vi "Obtain Request Events.vi"(8 "error in (no error)":errorcluster, 10 "Create New? (F)":bool) -> (0 "error out":errorcluster, 2 "Navigation Request Events":T1)   [LabVIEW 2022 SP3, in "Navigation.lvlib"]
doc: "This VI Obtains/Creates the Requests events that will be used for other modules to communicate with the module that owns this VI. These Requests events will be accessed only via Public API methods for this module.\n\n<b>NOTE</b>: The contents of this VI are automatically generated and modified by the <b>Tools > Delacor > DQMH</b> utilities. Consider using those utilities instead of making your own modifications to this VI.\n____\nHAMPEL SOFTWARE ENGINEERING v2.6.0 (2023-12-19 10:54)"
uses:
  Navigation.lvlib
  Request Events--cluster.ctl
  Stop Argument--cluster.ctl
  Show Panel Argument--cluster.ctl
  Hide Panel Argument--cluster.ctl
  Get Module Execution Status Argument--cluster.ctl
  Show Diagram Argument--cluster.ctl
  Prepare Argument--cluster.ctl
  Update Navigation Argument--cluster.ctl
  Sub-VIs/Ctl Target.ctl
  Configure Argument--cluster.ctl
  Select Listbox Element Argument--cluster.ctl
  Set Visibility Argument--cluster.ctl
  Sub-VIs/Visibility options--enum.ctl
  Set Disabled State Argument--cluster.ctl
panel:
  # "NOTE: The contents of this VI are automatically generated and modified by the Tools > Delacor > DQMH utilities. Consider using those utilities instead of making your own modifications to this VI."
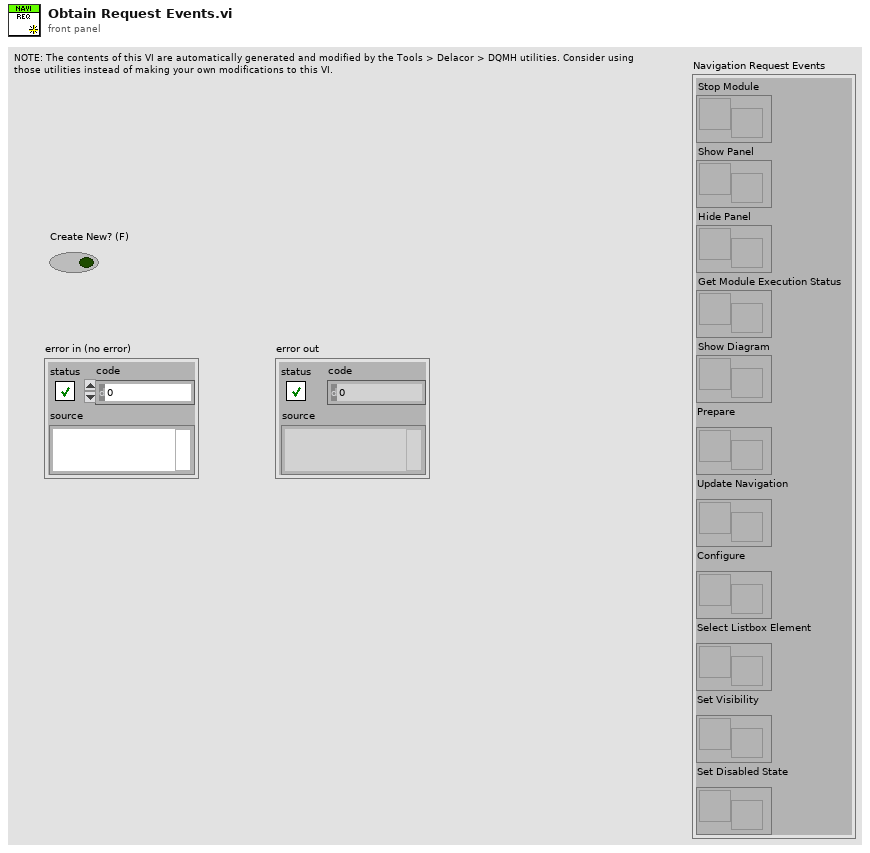
[diagram p1: front panel]
types:
  T1 = typedef "Navigation.lvlib/Request Events--cluster.ctl" = cluster{"Stop Module":refnum<user-event>, "Show Panel":refnum<user-event>, "Hide Panel":refnum<user-event>, "Get Module Execution Status":refnum<user-event>, "Show Diagram":refnum<user-event>, "Prepare":refnum<user-event>, "Update Navigation":refnum<user-event>, "Configure":refnum<user-event>, "Select Listbox Element":refnum<user-event>, "Set Visibility":refnum<user-event>, "Set Disabled State":refnum<user-event>}
  T2 = typedef "Navigation.lvlib/Set Disabled State Argument--cluster.ctl" = cluster{"Control Name":string, "Control State":enum8{"Enabled", "Disabled", "Disabled and Grayed Out"}}
  T3 = typedef "Navigation.lvlib/Set Visibility Argument--cluster.ctl" = cluster{"Control Name":string, "Visibility":T4}
  T4 = typedef "Navigation.lvlib/Visibility options--enum.ctl" = enum16{"visible", "hidden"}
  T5 = typedef "Navigation.lvlib/Select Listbox Element Argument--cluster.ctl" = cluster{"Name":string, "Index":i32}
  T6 = typedef "Navigation.lvlib/Configure Argument--cluster.ctl" = cluster{"Boolean":bool}
  T7 = typedef "Navigation.lvlib/Update Navigation Argument--cluster.ctl" = cluster{"Ctl Target":T8, "Name":string, "Data":variant}
  T8 = typedef "Navigation.lvlib/Ctl Target.ctl" = enum16{"Top Button", "Sub ListBox"}
  T9 = typedef "Navigation.lvlib/Prepare Argument--cluster.ctl" = cluster{"Boolean":bool}
  T10 = typedef "Navigation.lvlib/Hide Panel Argument--cluster.ctl" = cluster{"Hide Panel?":bool}
  T11 = typedef "Navigation.lvlib/Show Panel Argument--cluster.ctl" = cluster{"Show Panel?":bool}
  T12 = typedef "Navigation.lvlib/Show Diagram Argument--cluster.ctl" = cluster{"Debug?":bool}
  T13 = typedef "Navigation.lvlib/Get Module Execution Status Argument--cluster.ctl" = cluster{"Running?":bool}
  T14 = typedef "Navigation.lvlib/Stop Argument--cluster.ctl" = cluster{"Origin":string, "Exit via Stop Module Req?":bool, "Wait for Module to stop?":bool}
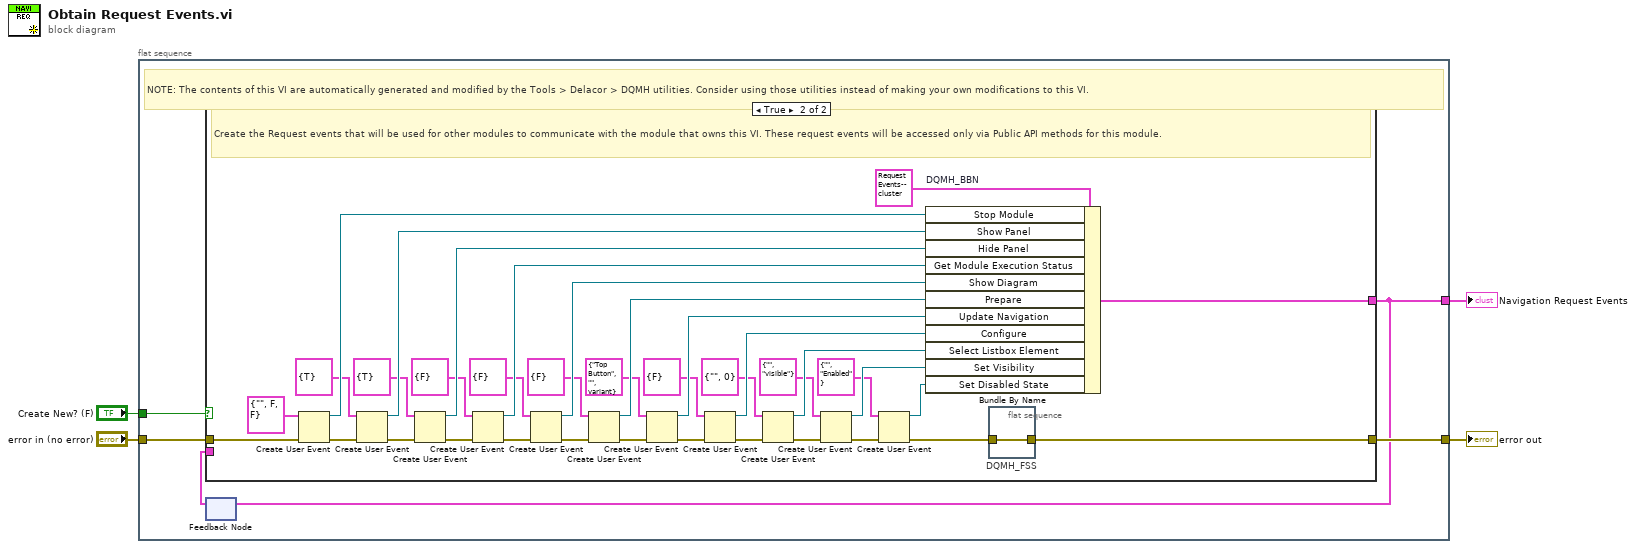
[diagram p0: block diagram]
diagram:
  n1 = flat-sequence {
    tunnel: [w9] -> w4
    tunnel: "error in (no error)" -> [w8]
    tunnel: [w6] -> w2
    tunnel: "Create New? (F)" -> [w5]
    frame #0 {
      # "NOTE: The contents of this VI are automatically generated and modified by the Tools > Delacor > DQMH utilities. Consider using those utilities instead of making your own modifications to this VI."
      n2 = feedback #1() -> (w7:T1)  [unwired: 1 in]
      n3 = case shown="True" w5 {
        tunnel: [w10 w38] -> w9
        tunnel: w8 -> [w10 w48]
        tunnel: [w11 w45] -> w6
        tunnel: w7 -> [w11 _]
        frame False {
          # "Obtain the Request events that were created in a previous call to this VI."
        }
        frame True {
          # "Create the Request events that will be used for other modules to communicate with the module that owns this VI. These request events will be accessed only via Public API methods for this module."
          n4 = Create User Event(user event datatype=T14 {"Origin"="", "Exit via Stop Module Req?"=FALSE, "Wait for Module to stop?"=FALSE} ("Stop Argument"), error in=w48) -> (user event=w46:refnum<user-event>, error out=w43:errorcluster)
          n5 = Create User Event(user event datatype=T11 {"Show Panel?"=TRUE} ("Show Panel Argument"), error in=w43) -> (user event=w42:refnum<user-event>, error out=w41:errorcluster)
          n6 = Create User Event(user event datatype=T10 {"Hide Panel?"=TRUE} ("Hide Panel Argument"), error in=w41) -> (user event=w40:refnum<user-event>, error out=w39:errorcluster)
          n7 = Create User Event(user event datatype=T13 {"Running?"=FALSE} ("Get Module Execution Status Argument"), error in=w39) -> (user event=w36:refnum<user-event>, error out=w37:errorcluster)
          n8 = Create User Event(user event datatype=T12 {"Debug?"=FALSE} ("Show Diagram Argument"), error in=w37) -> (user event=w33:refnum<user-event>, error out=w34:errorcluster)
          n9 = Create User Event(user event datatype=T9 {"Boolean"=FALSE} ("Prepare Argument"), error in=w34) -> (user event=w28:refnum<user-event>, error out=w29:errorcluster)
          n10 = Create User Event(user event datatype=T7 {"Ctl Target"=enum."Top Button", "Name"="", "Data"=variant} ("Update Navigation Argument"), error in=w29) -> (user event=w25:refnum<user-event>, error out=w26:errorcluster)
          n11 = Create User Event(user event datatype=T6 {"Boolean"=FALSE} ("Configure Argument"), error in=w26) -> (user event=w22:refnum<user-event>, error out=w23:errorcluster)
          n12 = Create User Event(user event datatype=T5 {"Name"="", "Index"=0} ("Select Listbox Element Argument"), error in=w23) -> (user event=w19:refnum<user-event>, error out=w20:errorcluster)
          n13 = Create User Event(user event datatype=T3 {"Control Name"="", "Visibility"=enum."visible"} ("Set Visibility Argument"), error in=w20) -> (user event=w16:refnum<user-event>, error out=w17:errorcluster)
          n14 = Create User Event(user event datatype=T2 {"Control Name"="", "Control State"=enum."Enabled"} ("Set Disabled State Argument"), error in=w17) -> (user event=w13:refnum<user-event>, error out=w14:errorcluster)
          n15 = Bundle By Name "DQMH_BBN"(cluster=T1 {"Stop Module"=refnum, "Show Panel"=refnum, "Hide Panel"=refnum, "Get Module Execution Status"=refnum, "Show Diagram"=refnum, "Prepare"=refnum, "Update Navigation"=refnum, "Configure"=refnum, "Select Listbox Element"=refnum, "Set Visibility"=refnum, "Set Disabled State"=refnum} ("output cluster"), "Stop Module"=w46, "Show Panel"=w42, "Hide Panel"=w40, "Get Module Execution Status"=w36, "Show Diagram"=w33, "Prepare"=w28, "Update Navigation"=w25, "Configure"=w22, "Select Listbox Element"=w19, "Set Visibility"=w16, "Set Disabled State"=w13) -> (w45:T1)
          n16 = flat-sequence "DQMH_FSS" {
            tunnel: w14 -> [w49]
            tunnel: [w49] -> w38
            frame #0 {
            }
          }
        }
      }
      n17 = feedback-in #1(w6) -> ()
    }
  }
  "Navigation Request Events" <- w2
  "error out" <- w4
